vi "From Variant.vi"(8 "error in (no error)":errorcluster, 10 "Variant":variant) -> (0 "error out":errorcluster, 3 "JSON Value out":refnum<class "JSON Value.lvclass">)   [LabVIEW 2016, in "JSFL Variant Support.lvlib"]
doc: "Creates a new JSON instance of the given type specified by the variant."
uses:
  JSFL Variant Support.lvlib
  JSON Value.lvclass
  New JSON Value/New JSON (String).vi
  <vilib>/Utility/Data Type/NI_Data Type.lvlib
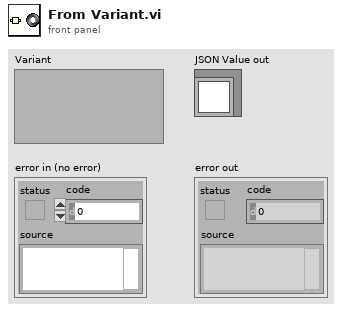
[diagram p1: front panel]
types:
  T1 = typedef "NI_Data Type.lvlib/Data Type.ctl" = enum8{"Invalid Type", "Void", "I8", "I16", "I32", "I64", "U8", "U16", "U32", "U64", "Single Float", "Double Float", "Extended Float", "Single Complex", "Double Complex", "Extended Complex", "Enum U8", "Enum U16", "Enum U32", "Enum U64", "Single Float With Unit", "Double Float With Unit", "Extended Float With Unit", "Single Complex with Unit", "Double Complex with Unit", "Extended Complex with Unit", "Boolean", "String", "Path", "Picture", "Tag", "Array", "Cluster", "Variant", "LV Variant", "Waveform", "Timestamp", "Digital Waveform", "Digital Data", "ExpressData", "Refnum", "External Data", "VI", "Poly VI", "LabVIEW Class Instance", "Fixed Point"}
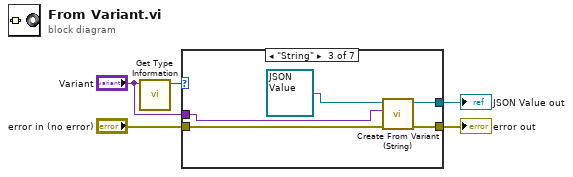
[diagram p0: block diagram]
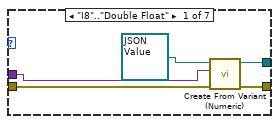
[diagram p2: hidden frame]
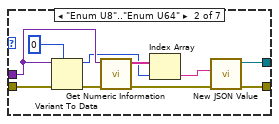
[diagram p3: hidden frame]
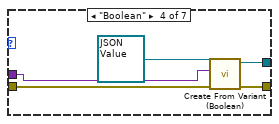
[diagram p4: hidden frame]
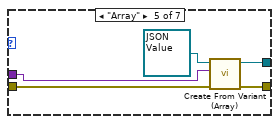
[diagram p5: hidden frame]
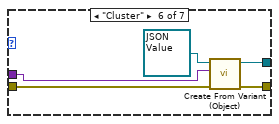
[diagram p6: hidden frame]
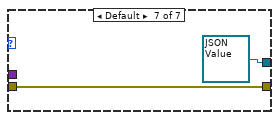
[diagram p7: hidden frame]
diagram:
  n1 = call <vilib>:"Get Type Information.vi"("Variant"="Variant") -> ("Type"=w5:T1)  [unwired: 6 in, 4 out]
  n2 = case shown="\"String\"" w5 {
    tunnel: "Variant" -> [w10 w18 w25 w30 w35 w40 _]
    tunnel: [w7 w20 w22 w27 w34 w37 refnum<class "JSON Value.lvclass"> refnum ("JSON out")] -> w1
    tunnel: "error in (no error)" -> [w9 w13 w24 w29 w33 w39 w42]
    tunnel: [w8 w19 w23 w28 w32 w38 w42] -> w2
    frame "I8".."Double Float" {
      n3 = call "Create From Variant (Numeric).vi"("error in (no error)"=w9, "Variant"=w10, "JSON Numeric in"=refnum<class "JSON Value.lvclass"> refnum ("JSON out")) -> ("error out"=w8:errorcluster, "JSON Numeric out"=w7:refnum<class "JSON Value.lvclass">)  [unwired: 7 in]
    }
    frame "Enum U8".."Enum U64" {
      n4 = Variant To Data(error in=w13, type=u64 0, Variant=w18) -> (data=w15:u64, error out=w12:errorcluster)
      n5 = call <vilib>:"Get Numeric Information.vi"("error in (no error)"=w12, "Variant"=w18) -> ("error out"=w11:errorcluster, "Enum Names"=w16:string[])  [unwired: 6 in, 2 out]
      n6 = Index Array(array=w16, index=w15) -> (element=w14:string)
      n7 = call-poly "New JSON Value.vi"("error in (no error)"=w11, "value"=w14) -> ("error out"=w19:errorcluster, "JSON Value out"=w20:refnum<class "JSON Value.lvclass">)  [unwired: 8 in]
    }
    frame "String" {
      n8 = call "Create From Variant (String).vi"("error in (no error)"=w24, "Variant"=w25, "JSON String in"=refnum<class "JSON Value.lvclass"> refnum ("JSON out")) -> ("error out"=w23:errorcluster, "JSON String out"=w22:refnum<class "JSON Value.lvclass">)  [unwired: 7 in]
    }
    frame "Boolean" {
      n9 = call "Create From Variant (Boolean).vi"("error in (no error)"=w29, "Variant"=w30, "JSON Boolean in"=refnum<class "JSON Value.lvclass"> refnum ("JSON out")) -> ("error out"=w28:errorcluster, "JSON Boolean out"=w27:refnum<class "JSON Value.lvclass">)  [unwired: 7 in]
    }
    frame "Array" {
      n10 = call "Create From Variant (Array).vi"("error in (no error)"=w33, "Variant"=w35, "JSON Value in"=refnum<class "JSON Value.lvclass"> refnum ("JSON Array in")) -> ("error out"=w32:errorcluster, "JSON Value out"=w34:refnum<class "JSON Value.lvclass">)  [unwired: 7 in]
    }
    frame "Cluster" {
      n11 = call "Create From Variant (Object).vi"("error in (no error)"=w39, "Variant"=w40, "JSON Value in"=refnum<class "JSON Value.lvclass"> refnum ("JSON Array in")) -> ("error out"=w38:errorcluster, "JSON Value out"=w37:refnum<class "JSON Value.lvclass">)  [unwired: 7 in]
    }
    frame Default {
    }
  }
  "error out" <- w2
  "JSON Value out" <- w1
